vi "HelloWorld.vi"   [LabVIEW 2024]
uses:
  SDL3/Video/WindowFlags--ring.ctl
  SDL3/Pixels/PixelFormat--enum.ctl
  SDL3/Render/TextureAccess-enum.ctl
  SDL3/Init/InitFlags--ring.ctl
  SDL3/Events/MouseMotionEvent--cluster.ctl
  SDL3/Video/WindowID--integer.ctl
  SDL3/Mouse/MouseID--integer.ctl
  SDL3/Mouse/MouseButtonFlags--ring.ctl
  SDL3/Init/Init.lvlib
  SDL3/Video/Video.lvlib
  SDL3/Render/Render.lvlib
  SDL3/Pixels/Pixels.lvlib
  SDL3/Timer/Timer.lvlib
  SDL3/Events/Events.lvlib
  SDL3/Mouse/Mouse.lvlib
types:
  T1 = typedef "SDL3.lvlib/Events.lvlib/MouseMotionEvent--cluster.ctl" = cluster{"timestamp":u64, "windowID":T2, "which":T3, "state":T4, "x":sgl, "y":sgl, "xrel":sgl, "yrel":sgl}
  T2 = typedef "SDL3.lvlib/Video.lvlib/WindowID--integer.ctl" = u32
  T3 = typedef "SDL3.lvlib/Mouse.lvlib/MouseID--integer.ctl" = u32
  T4 = typedef "SDL3.lvlib/Mouse.lvlib/MouseButtonFlags--ring.ctl" = u32
  T5 = typedef "SDL3.lvlib/Init.lvlib/InitFlags--ring.ctl" = u32
  T6 = enum32{"Invalid", "Standard", "Closed", "Hidden", "Minimized", "Maximized"}
  T7 = typedef "SDL3.lvlib/Render.lvlib/TextureAccess-enum.ctl" = enum32{"SDL_TEXTUREACCESS_STATIC", "SDL_TEXTUREACCESS_STREAMING", "SDL_TEXTUREACCESS_TARGET"}
  T8 = typedef "SDL3.lvlib/Pixels.lvlib/PixelFormat--enum.ctl" = enum32{"SDL_PIXELFORMAT_UNKNOWN", "SDL_PIXELFORMAT_INDEX1LSB", "SDL_PIXELFORMAT_INDEX1MSB", "SDL_PIXELFORMAT_INDEX2LSB", "SDL_PIXELFORMAT_INDEX2MSB", "SDL_PIXELFORMAT_INDEX4LSB", "SDL_PIXELFORMAT_INDEX4MSB", "SDL_PIXELFORMAT_INDEX8", "SDL_PIXELFORMAT_RGB332", "SDL_PIXELFORMAT_XRGB4444", "SDL_PIXELFORMAT_XBGR4444", "SDL_PIXELFORMAT_XRGB1555", "SDL_PIXELFORMAT_XBGR1555", "SDL_PIXELFORMAT_ARGB4444", "SDL_PIXELFORMAT_RGBA4444", "SDL_PIXELFORMAT_ABGR4444", "SDL_PIXELFORMAT_BGRA4444", "SDL_PIXELFORMAT_ARGB1555", "SDL_PIXELFORMAT_RGBA5551", "SDL_PIXELFORMAT_ABGR1555", "SDL_PIXELFORMAT_BGRA5551", "SDL_PIXELFORMAT_RGB565", "SDL_PIXELFORMAT_BGR565", "SDL_PIXELFORMAT_RGB24", "SDL_PIXELFORMAT_BGR24", "SDL_PIXELFORMAT_XRGB8888", "SDL_PIXELFORMAT_RGBX8888", "SDL_PIXELFORMAT_XBGR8888", "SDL_PIXELFORMAT_BGRX8888", "SDL_PIXELFORMAT_ARGB8888", "SDL_PIXELFORMAT_RGBA8888", "SDL_PIXELFORMAT_ABGR8888", "SDL_PIXELFORMAT_BGRA8888", "SDL_PIXELFORMAT_XRGB2101010", "SDL_PIXELFORMAT_XBGR2101010", "SDL_PIXELFORMAT_ARGB2101010", "SDL_PIXELFORMAT_ABGR2101010", "SDL_PIXELFORMAT_RGB48", "SDL_PIXELFORMAT_BGR48", "SDL_PIXELFORMAT_RGBA64", "SDL_PIXELFORMAT_ARGB64", "SDL_PIXELFORMAT_BGRA64", "SDL_PIXELFORMAT_ABGR64", "SDL_PIXELFORMAT_RGB48_FLOAT", "SDL_PIXELFORMAT_BGR48_FLOAT", "SDL_PIXELFORMAT_RGBA64_FLOAT", "SDL_PIXELFORMAT_ARGB64_FLOAT", "SDL_PIXELFORMAT_BGRA64_FLOAT", "SDL_PIXELFORMAT_ABGR64_FLOAT", "SDL_PIXELFORMAT_RGB96_FLOAT", "SDL_PIXELFORMAT_BGR96_FLOAT", "SDL_PIXELFORMAT_RGBA128_FLOAT", "SDL_PIXELFORMAT_ARGB128_FLOAT", "SDL_PIXELFORMAT_BGRA128_FLOAT", "SDL_PIXELFORMAT_ABGR128_FLOAT", "SDL_PIXELFORMAT_YV12", "SDL_PIXELFORMAT_IYUV", "SDL_PIXELFORMAT_YUY2", "SDL_PIXELFORMAT_UYVY", "SDL_PIXELFORMAT_YVYU", "SDL_PIXELFORMAT_NV12", "SDL_PIXELFORMAT_NV21", "SDL_PIXELFORMAT_P010", "SDL_PIXELFORMAT_EXTERNAL_OES"}
  T9 = typedef "SDL3.lvlib/Video.lvlib/WindowFlags--ring.ctl" = u64
  T10 = typedef "SDL3.lvlib/Events.lvlib/EventType--enum.ctl" = enum16{"LV_NONE", "LV_UNSUPPORTED", "SDL_EVENT_QUIT", "SDL_EVENT_LOCALE_CHANGED", "SDL_EVENT_SYSTEM_THEME_CHANGED", "SDL_EVENT_DISPLAY_ORIENTATION", "SDL_EVENT_DISPLAY_ADDED", "SDL_EVENT_DISPLAY_REMOVED", "SDL_EVENT_DISPLAY_MOVED", "SDL_EVENT_DISPLAY_DESKTOP_MODE_CHANGED", "SDL_EVENT_DISPLAY_CURRENT_MODE_CHANGED", "SDL_EVENT_DISPLAY_CONTENT_SCALE_CHANGED", "SDL_EVENT_WINDOW_SHOWN", "SDL_EVENT_WINDOW_HIDDEN", "SDL_EVENT_WINDOW_EXPOSED", "SDL_EVENT_WINDOW_MOVED", "SDL_EVENT_WINDOW_RESIZED", "SDL_EVENT_WINDOW_PIXEL_SIZE_CHANGED", "SDL_EVENT_WINDOW_METAL_VIEW_RESIZED", "SDL_EVENT_WINDOW_MINIMIZED", "SDL_EVENT_WINDOW_MAXIMIZED", "SDL_EVENT_WINDOW_RESTORED", "SDL_EVENT_WINDOW_MOUSE_ENTER", "SDL_EVENT_WINDOW_MOUSE_LEAVE", "SDL_EVENT_WINDOW_FOCUS_GAINED", "SDL_EVENT_WINDOW_FOCUS_LOST", "SDL_EVENT_WINDOW_CLOSE_REQUESTED", "SDL_EVENT_WINDOW_HIT_TEST", "SDL_EVENT_WINDOW_ICCPROF_CHANGED", "SDL_EVENT_WINDOW_DISPLAY_CHANGED", "SDL_EVENT_WINDOW_DISPLAY_SCALE_CHANGED", "SDL_EVENT_WINDOW_SAFE_AREA_CHANGED", "SDL_EVENT_WINDOW_OCCLUDED", "SDL_EVENT_WINDOW_ENTER_FULLSCREEN", "SDL_EVENT_WINDOW_LEAVE_FULLSCREEN", "SDL_EVENT_WINDOW_DESTROYED", "SDL_EVENT_WINDOW_HDR_STATE_CHANGED", "SDL_EVENT_KEY_DOWN", "SDL_EVENT_KEY_UP", "SDL_EVENT_TEXT_EDITING", "SDL_EVENT_TEXT_INPUT", "SDL_EVENT_KEYMAP_CHANGED", "SDL_EVENT_KEYBOARD_ADDED", "SDL_EVENT_KEYBOARD_REMOVED", "SDL_EVENT_TEXT_EDITING_CANDIDATES", "SDL_EVENT_MOUSE_MOTION", "SDL_EVENT_MOUSE_BUTTON_DOWN", "SDL_EVENT_MOUSE_BUTTON_UP", "SDL_EVENT_MOUSE_WHEEL", "SDL_EVENT_MOUSE_ADDED", "SDL_EVENT_MOUSE_REMOVED", "SDL_EVENT_JOYSTICK_AXIS_MOTION", "SDL_EVENT_JOYSTICK_BALL_MOTION", "SDL_EVENT_JOYSTICK_HAT_MOTION", "SDL_EVENT_JOYSTICK_BUTTON_DOWN", "SDL_EVENT_JOYSTICK_BUTTON_UP", "SDL_EVENT_JOYSTICK_ADDED", "SDL_EVENT_JOYSTICK_REMOVED", "SDL_EVENT_JOYSTICK_BATTERY_UPDATED", "SDL_EVENT_JOYSTICK_UPDATE_COMPLETE", "SDL_EVENT_GAMEPAD_AXIS_MOTION", "SDL_EVENT_GAMEPAD_BUTTON_DOWN", "SDL_EVENT_GAMEPAD_BUTTON_UP", "SDL_EVENT_GAMEPAD_ADDED", "SDL_EVENT_GAMEPAD_REMOVED", "SDL_EVENT_GAMEPAD_REMAPPED", "SDL_EVENT_GAMEPAD_TOUCHPAD_DOWN", "SDL_EVENT_GAMEPAD_TOUCHPAD_MOTION", "SDL_EVENT_GAMEPAD_TOUCHPAD_UP", "SDL_EVENT_GAMEPAD_SENSOR_UPDATE", "SDL_EVENT_GAMEPAD_UPDATE_COMPLETE", "SDL_EVENT_GAMEPAD_STEAM_HANDLE_UPDATED", "SDL_EVENT_FINGER_DOWN", "SDL_EVENT_FINGER_UP", "SDL_EVENT_FINGER_MOTION", "SDL_EVENT_CLIPBOARD_UPDATE", "SDL_EVENT_DROP_FILE", "SDL_EVENT_DROP_TEXT", "SDL_EVENT_DROP_BEGIN", "SDL_EVENT_DROP_COMPLETE", "SDL_EVENT_DROP_POSITION", "SDL_EVENT_AUDIO_DEVICE_ADDED", "SDL_EVENT_AUDIO_DEVICE_REMOVED", "SDL_EVENT_AUDIO_DEVICE_FORMAT_CHANGED", "SDL_EVENT_SENSOR_UPDATE", "SDL_EVENT_PEN_PROXIMITY_IN", "SDL_EVENT_PEN_PROXIMITY_OUT", "SDL_EVENT_PEN_DOWN", "SDL_EVENT_PEN_UP", "SDL_EVENT_PEN_BUTTON_DOWN", "SDL_EVENT_PEN_BUTTON_UP", "SDL_EVENT_PEN_MOTION", "SDL_EVENT_PEN_AXIS", "SDL_EVENT_CAMERA_DEVICE_ADDED", "SDL_EVENT_CAMERA_DEVICE_REMOVED", "SDL_EVENT_CAMERA_DEVICE_APPROVED", "SDL_EVENT_CAMERA_DEVICE_DENIED", "SDL_EVENT_RENDER_TARGETS_RESET", "SDL_EVENT_RENDER_DEVICE_RESET", "SDL_EVENT_POLL_SENTINEL", "SDL_EVENT_USER"}
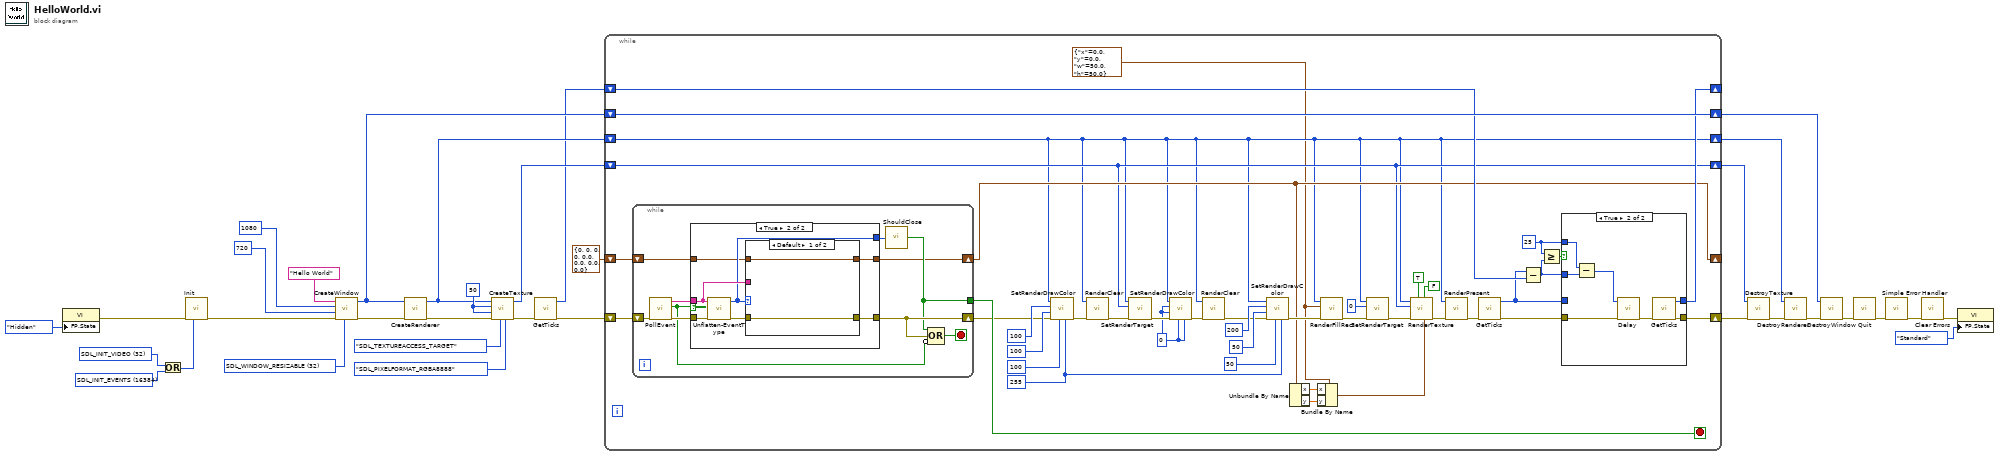
[diagram p0: block diagram]
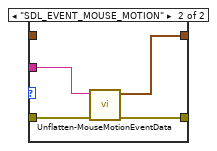
[diagram p3: hidden frame]
diagram:
  w2 = T5 16384 items=["NONE"=0, "SDL_INIT_AUDIO"=16, "SDL_INIT_VIDEO"=32, "SDL_INIT_JOYSTICK"=512, "SDL_INIT_HAPTIC"=4096, "SDL_INIT_GAMEPAD"=8192, "SDL_INIT_EVENTS"=16384, "SDL_INIT_SENSOR"=32768, "SDL_INIT_CAMER"=65536] ("y")
  w7 = T5 32 items=["NONE"=0, "SDL_INIT_AUDIO"=16, "SDL_INIT_VIDEO"=32, "SDL_INIT_JOYSTICK"=512, "SDL_INIT_HAPTIC"=4096, "SDL_INIT_GAMEPAD"=8192, "SDL_INIT_EVENTS"=16384, "SDL_INIT_SENSOR"=32768, "SDL_INIT_CAMER"=65536] ("InitFlags")
  w25 = 50 ("w")
  w30 = T9 32 items=["0"=0, "SDL_WINDOW_FULLSCREEN"=1, "SDL_WINDOW_OPENGL"=2, "SDL_WINDOW_OCCLUDED"=4, "SDL_WINDOW_HIDDEN"=8, "SDL_WINDOW_BORDERLESS"=16, "SDL_WINDOW_RESIZABLE"=32, "SDL_WINDOW_MINIMIZED"=64, "SDL_WINDOW_MAXIMIZED"=128, "SDL_WINDOW_MOUSE_GRABBED"=256, "SDL_WINDOW_INPUT_FOCUS"=512, "SDL_WINDOW_MOUSE_FOCUS"=1024, "SDL_WINDOW_EXTERNAL"=2048, "SDL_WINDOW_MODAL"=4096, "SDL_WINDOW_HIGH_PIXEL_DENSITY"=8192, "SDL_WINDOW_MOUSE_CAPTURE"=16384, "SDL_WINDOW_MOUSE_RELATIVE_MODE"=32768, "SDL_WINDOW_ALWAYS_ON_TOP"=65536, "SDL_WINDOW_UTILITY"=131072, "SDL_WINDOW_TOOLTIP"=262144, "SDL_WINDOW_POPUP_MENU"=524288, "SDL_WINDOW_KEYBOARD_GRABBED"=1048576, "SDL_WINDOW_VULKAN"=268435456, "SDL_WINDOW_METAL"=536870912, "SDL_WINDOW_TRANSPARENT"=1073741824, "SDL_WINDOW_NOT_FOCUSABLE"=2147483648] ("flags (0)")
  n1 = property class="VI"("FP.State"=T6."Hidden" ("Front Panel Window:State")) -> (error out=w12:errorcluster)  [unwired: 2 in, 1 out]
  n2 = Or(x=w7, y=w2) -> (x .or. y?=w3:T5)
  n3 = call "Init.vi"("InitFlags"=w3, "No Error"=w12) -> ("error out"=w33:errorcluster)  [unwired: 9 in]
  n4 = call "CreateWindow.vi"("flags (0)"=w30, "No Error"=w33, "h"=720, "w"=1080, "title"="Hello World") -> ("error out"=w29:errorcluster, "window [SDL_Window *]"=w21:i64)  [unwired: 5 in]
  n5 = call "CreateRenderer.vi"("No Error"=w29, "window [SDL_Window *]"=w21) -> ("Error Out"=w26:errorcluster, "renderer [SDL_Renderer *]"=w20:i64)  [unwired: 8 in]
  n6 = call "CreateTexture.vi"("pixel_format"=PixelFormat--enum."SDL_PIXELFORMAT_RGBA8888", "texture_access"=TextureAccess-enum."SDL_TEXTUREACCESS_TARGET", "No Error"=w26, "h"=w25, "w"=w25, "renderer [SDL_Renderer *]"=w20) -> ("error out"=w6:errorcluster, "texture [SDL_Texture *]"=w19:i64)  [unwired: 4 in]
  n7 = call "GetTicks.vi"("No Error"=w6) -> ("error out"=w5:errorcluster, "ticks [ms]"=w4:u64)  [unwired: 9 in]
  n8 = while {
    shift-right: [w42] -> w16
    shift-left: w19 -> [w42]
    shift-right: [w37] -> w17
    shift-left: w20 -> [w37]
    shift-right: [w74] -> w18
    shift-left: w21 -> [w74]
    shift-right: [w59] -> w28
    shift-left: w5 -> [w50]
    shift-right: [w58] -> _
    shift-left: w4 -> [w55]
    shift-right: [w47] -> _
    shift-left: T1 {"timestamp"=0, "windowID"=0, "which"=0, "state"=0, "x"=0.0, "y"=0.0, "xrel"=0.0, "yrel"=0.0} ("MouseMotionEvent") -> [w48]
    stop <- w49 stop-if-true
    w36 = u8 0 ("r")
    w54 = u64 25
    w34 = cluster{"x":sgl, "y":sgl, "w":sgl, "h":sgl} {"x"=0.0, "y"=0.0, "w"=50.0, "h"=50.0} ("rect")
    w39 = u8 255 ("a")
    n9 = while {
      shift-right: [w79] -> w44
      shift-left: w50 -> [w84]
      tunnel: [w77] -> w49
      shift-right: [w76] -> w47
      shift-left: w48 -> [w75]
      stop <- w83 stop-if-true
      n10 = call "PollEvent.vi"("No Error"=w84) -> ("error out"=w82:errorcluster, "Event Occured?"=w80:bool, "Event Binary Data"=w81:string)  [unwired: 8 in]
      n11 = case shown="True" w80 {
        tunnel: w82 -> [w86 w93]
        tunnel: w81 -> [_ w92]
        tunnel: [w86 w89] -> w79
        tunnel: [_ w91] -> w78
        tunnel: [w85 w88] -> w76
        tunnel: w75 -> [w85 w87]
        frame False {
        }
        frame True {
          n12 = call "Unflatten-EventType.vi"("error in (no error)"=w93, "Event Binary Data In"=w92) -> ("error out"=w90:errorcluster, "EventType"=w91:T10)  [unwired: 8 in]
          n13 = case shown="Default" w91 {
            tunnel: w92 -> [_ w98]
            tunnel: w90 -> [w95 w99]
            tunnel: [w95 w97] -> w89
            tunnel: [w94 w96] -> w88
            tunnel: w87 -> [w94 _]
            frame Default {
            }
            frame "SDL_EVENT_MOUSE_MOTION" {
              n14 = call "Unflatten-MouseMotionEventData.vi"("error in (no error)"=w99, "Event Binary Data"=w98) -> ("error out"=w97:errorcluster, "MouseMotionEvent"=w96:T1)  [unwired: 8 in]
            }
          }
        }
      }
      n15 = call "ShouldClose.vi"("EventType"=w78) -> ("Close?"=w77:bool)
      n16 = Compound Arithmetic op=OR(w77, w79, invert w80) -> (w83:bool)
    }
    n17 = call "SetRenderDrawColor.vi"("a"=w39, "b"=u8 100, "No Error"=w44, "g"=u8 100, "r"=u8 100, "renderer [SDL_Renderer *]"=w37) -> ("error out"=w71:errorcluster)  [unwired: 5 in]
    n18 = call "RenderClear.vi"("No Error"=w71, "renderer [SDL_Renderer *]"=w37) -> ("error out"=w43:errorcluster)  [unwired: 9 in]
    n19 = call "SetRenderTarget.vi"("No Error"=w43, "texture [SDL_Texture *]"=w42, "renderer [SDL_Renderer *]"=w37) -> ("error out"=w41:errorcluster)  [unwired: 8 in]
    n20 = call "SetRenderDrawColor.vi"("a"=w36, "b"=w36, "No Error"=w41, "g"=w36, "r"=w36, "renderer [SDL_Renderer *]"=w37) -> ("error out"=w40:errorcluster)  [unwired: 5 in]
    n21 = call "RenderClear.vi"("No Error"=w40, "renderer [SDL_Renderer *]"=w37) -> ("error out"=w38:errorcluster)  [unwired: 9 in]
    n22 = call "SetRenderDrawColor.vi"("a"=w39, "b"=u8 50, "No Error"=w38, "g"=u8 50, "r"=u8 200, "renderer [SDL_Renderer *]"=w37) -> ("error out"=w64:errorcluster)  [unwired: 5 in]
    n23 = Unbundle By Name(w47) -> ("x"=w46:sgl, "y"=w45:sgl)
    n24 = Bundle By Name(cluster=w34, "x"=w46, "y"=w45) -> (w35:cluster{"x":sgl, "y":sgl, "w":sgl, "h":sgl})
    n25 = call "RenderFillRect.vi"("No Error"=w64, "rect"=w34, "renderer [SDL_Renderer *]"=w37) -> ("error out"=w60:errorcluster)  [unwired: 8 in]
    n26 = call "SetRenderTarget.vi"("No Error"=w60, "texture [SDL_Texture *]"=i64 0, "renderer [SDL_Renderer *]"=w37) -> ("error out"=w72:errorcluster)  [unwired: 8 in]
    n27 = call "RenderTexture.vi"("dstrect"=w35, "Entire Rendering Target (F)"=FALSE, "Entire Texture (F)"=TRUE, "No Error"=w72, "texture [SDL_Texture *]"=w42, "renderer [SDL_Renderer *]"=w37) -> ("error out"=w73:errorcluster)  [unwired: 5 in]
    n28 = call "RenderPresent.vi"("No Error"=w73, "renderer [SDL_Renderer *]"=w37) -> ("error out"=w57:errorcluster)  [unwired: 9 in]
    n29 = call "GetTicks.vi"("No Error"=w57) -> ("error out"=w56:errorcluster, "ticks [ms]"=w51:u64)  [unwired: 9 in]
    n30 = Subtract(x=w51, y=w55) -> (x-y=w53:u64)
    n31 = Greater Or Equal?(x=w54, y=w53) -> (x >= y?=w52:bool)
    n32 = case shown="True" w52 {
      tunnel: [w100 w108] -> w59
      tunnel: [w101 w107] -> w58
      tunnel: w56 -> [w100 w106]
      tunnel: w54 -> [_ w105]
      tunnel: w53 -> [_ w104]
      tunnel: w51 -> [w101 _]
      frame False {
      }
      frame True {
        n33 = Subtract(x=w105, y=w104) -> (x-y=w102:u64)
        n34 = call "Delay.vi"("No Error"=w106, "ms"=w102) -> ("error out"=w103:errorcluster)  [unwired: 9 in]
        n35 = call "GetTicks.vi"("No Error"=w103) -> ("error out"=w108:errorcluster, "ticks [ms]"=w107:u64)  [unwired: 9 in]
      }
    }
  }
  n36 = call "DestroyTexture.vi"("No Error"=w28, "texture [SDL_Texture *]"=w16) -> ("error out"=w22:errorcluster)  [unwired: 9 in]
  n37 = call "DestroyRenderer.vi"("No Error"=w22, "renderer [SDL_Renderer *]"=w17) -> ("error out"=w27:errorcluster)  [unwired: 9 in]
  n38 = call "DestroyWindow.vi"("No Error"=w27, "window [SDL_Window*]"=w18) -> ("error out"=w32:errorcluster)  [unwired: 9 in]
  n39 = call "Quit.vi"("No Error"=w32) -> ("error out"=w10:errorcluster)  [unwired: 10 in]
  n40 = call <vilib>:"Simple Error Handler.vi"("error in (no error)"=w10) -> ("error out"=w9:errorcluster)  [unwired: 4 in, 4 out]
  n41 = call <vilib>:"Clear Errors.vi"("error in (no error)"=w9) -> ("error out"=w8:errorcluster)  [unwired: 5 in, 1 out]
  n42 = property class="VI"(error in=w8, "FP.State"=T6."Standard" ("Front Panel Window:State")) -> ()  [unwired: 1 in, 2 out]
